vi "LVFunction_Imop_Compute_MTF from HasoField.vi"(0 "Path":path, 5 "SurfaceFloat.lvclass":refnum<class "SurfaceFloat.lvclass">, 7 "SurfaceFloat.lvclass":refnum<class "SurfaceFloat.lvclass">, 9 "Dimensions_µm":T1={"Size"={"X"=32, "Y"=32}, "Step"={"X"=1.0, "Y"=1.0}}, 11 "error in (no error)":errorcluster) -> (6 "SurfaceFloat.lvclass":refnum<class "SurfaceFloat.lvclass">, 8 "SurfaceFloat.lvclass":refnum<class "SurfaceFloat.lvclass">, 15 "error out":errorcluster)   [LabVIEW 2020]
doc: "Modulation transfer function from point spread function surface.\n\n--------------------------------------------------------------------------------\n\n<B>surface_with_pupil_psfIn</B> : PSF stored as cSurface.\n\n<B>surface_with_pupil_psfOut</B> : PSF stored as cSurface.\n\n<B>config_file_path</B> : Absolute path to the Haso configuration file.\n\n<B>SurfaceMTF</B> : MTF stored as cSurface.\n\n<B>ErrorIn</B> : Error\n\n<B>ErrorOut</B> : Error"
uses:
  General dimensions definition.ctl
  Point2D.ctl
  Point2Df.ctl
  SurfaceFloat.lvclass
  LVClasse_SurfaceFloat Read SurfaceFloat.vi
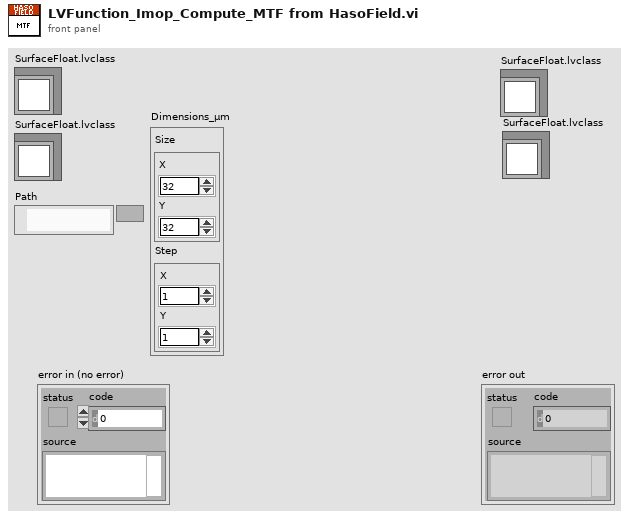
[diagram p1: front panel]
types:
  T1 = typedef "General dimensions definition.ctl" = cluster{"Size":T2, "Step":T3}
  T2 = typedef "Point2D.ctl" = cluster{"X":u32, "Y":u32}
  T3 = typedef "Point2Df.ctl" = cluster{"X":sgl, "Y":sgl}
  T4 = typedef "ClassID.ctl" = i64
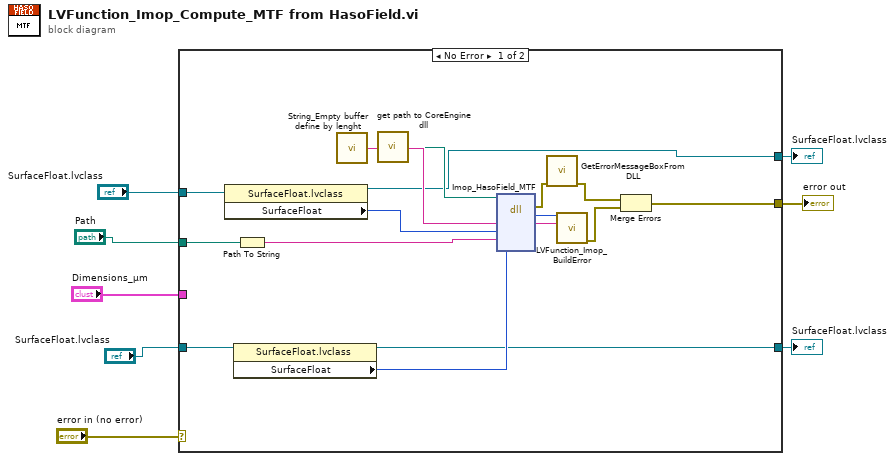
[diagram p0: block diagram]
diagram:
  n1 = case shown="No Error" "error in (no error)" {
    selector: "error in (no error)" -> [_ w27]
    tunnel: [w17 w27] -> w7
    tunnel: "Path" -> [w16 _]
    tunnel: "Dimensions_µm" -> [_ _]
    tunnel: "SurfaceFloat.lvclass" -> [w14 w26]
    tunnel: "SurfaceFloat.lvclass" -> [w13 w25]
    tunnel: [w9 w26] -> w2
    tunnel: [w10 w25] -> w1
    frame No Error {
      n2 = property class="SurfaceFloat.lvclass"(reference=w14) -> (reference out=w9:refnum<class "SurfaceFloat.lvclass">, "SurfaceFloat"=w11:T4)  [unwired: 1 in, 1 out]
      n3 = property class="SurfaceFloat.lvclass"(reference=w13) -> (reference out=w10:refnum<class "SurfaceFloat.lvclass">, "SurfaceFloat"=w12:T4)  [unwired: 1 in, 1 out]
      n4 = Path To String(path=w16) -> (string=w15:string)
      n5 = call "String_Empty buffer define by lenght.vi"() -> ("Empty buffer"=w24:string)  [unwired: 1 in]
      n6 = call "get path to CoreEngine dll.vi"() -> ("path to wavekit library"=w21:path)  [unwired: 14 in, 1 out]
      n7 = dll-call lib="D:/2_trunk/Soft_haso/ImOpCoreEngine4_LV2011/DLLs/ImopEngine4_vc100.dll" fn="Imop_HasoField_MTF"(path in=w21, "message"=w24, "surface_with_pupil_psf"=w11, "config_file_path"=w15, "surface_with_pupil_mtf"=w12) -> (error out=w20:errorcluster, "return type"=w22:i32, "message"=w23:string)  [unwired: 5 in, 1 out]
      n8 = call "GetErrorMessageBoxFromDLL.vi"("error IN"=w20) -> ("error OUT"=w19:errorcluster)  [unwired: 10 in]
      n9 = call "LVFunction_Imop_BuildError.vi"("code"=w22, "String to Prepend to source (\"\")"=w23) -> ("error out"=w18:errorcluster)  [unwired: 13 in]
      n10 = Merge Errors(w19, w18) -> (w17:errorcluster)
    }
    frame Error {
    }
  }
  "error out" <- w7
  "SurfaceFloat.lvclass" <- w2
  "SurfaceFloat.lvclass" <- w1
